vi "Configure Trigger (ZONE).vi"(4 "Enable Zone Qualified Trigger (F: Disable)":bool, 5 "Size and Location of Zone":T1={"Width of Zone (0 s)"=0.0, "Height of Zone (0 v)"=0.0, "X Center of Zone (0.0001 s)"=0.0001, "Y Center of Zone (0 v)"=5.0}, 6 "Zone State (F: Disable)":bool, 7 "Qualifying Condition (0: Must Intersect)":i32(ring) items=["Must Intersect", "Must Not Intersect"], 8 "error in (no error)":errorcluster, 9 "Zone Number (1: Zone 1)":i32(ring)=1 items=["Zone 1"=1, "Zone 2"=2], 10 "Analog Source Channel (0: Channel 1)":i32(ring) items=["Channel 1", "Channel 2", "Channel 3", "Channel 4"], 11 "VISA resource name":refnum<visa-resource-name>) -> (0 "error out":errorcluster, 3 "VISA resource name out":refnum<visa-resource-name>)   [LabVIEW 2015, in "Agilent 2000 3000 X-Series.lvlib"]
doc: "Configures the zone trigger mode. \n\nNote(s):\nThis VI is only applicable for Agilent InfiniiVision 4000 X-Series and 3000 T X-Series Oscilloscopes."
uses:
  <instrlib>/Agilent 2000 3000 X-Series/Agilent 2000 3000 X-Series.lvlib
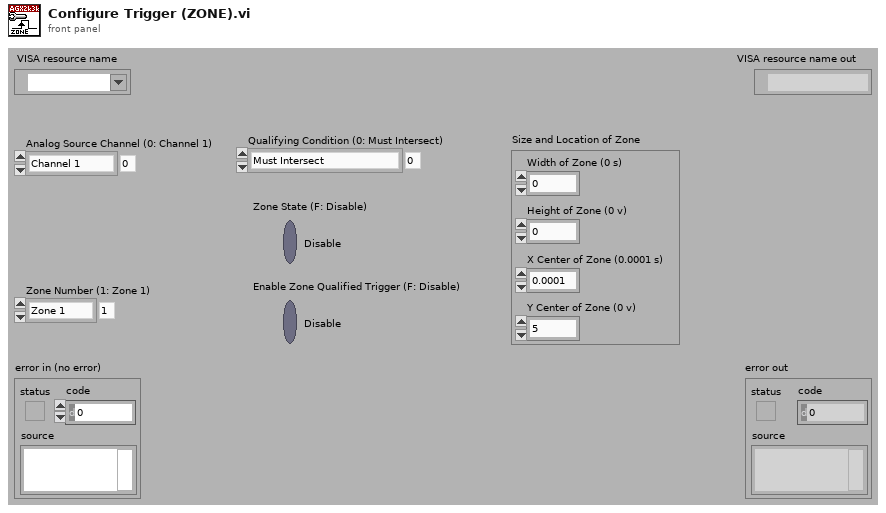
[diagram p1: front panel]
types:
  T1 = cluster{"Width of Zone (0 s)":dbl, "Height of Zone (0 v)":dbl, "X Center of Zone (0.0001 s)":dbl, "Y Center of Zone (0 v)":dbl}
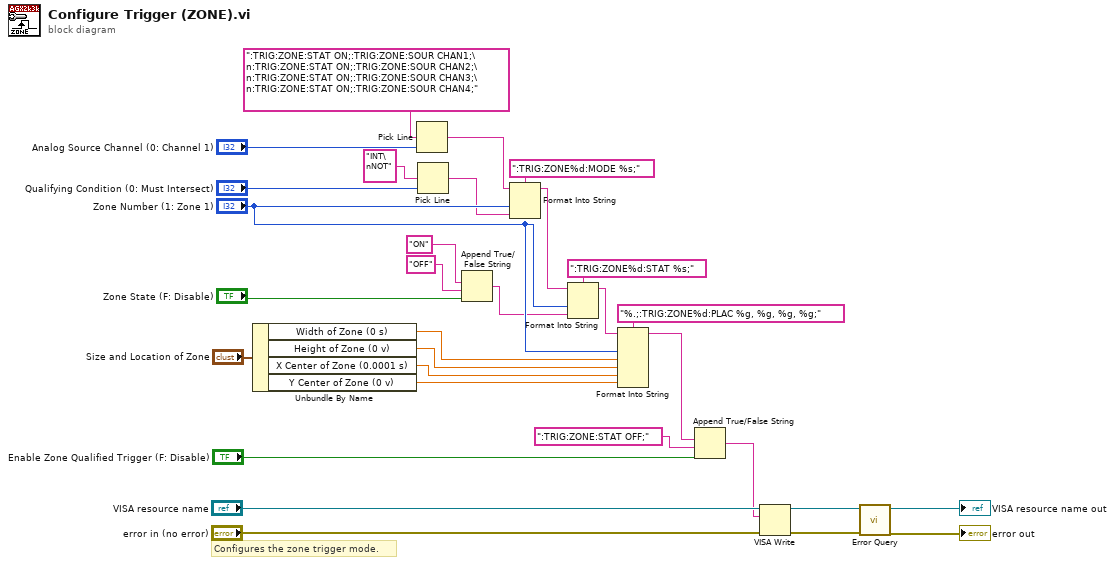
[diagram p0: block diagram]
diagram:
  # "Configures the zone trigger mode."
  n1 = Unbundle By Name("Size and Location of Zone") -> ("Width of Zone (0 s)"=w9:dbl, "Height of Zone (0 v)"=w8:dbl, "X Center of Zone (0.0001 s)"=w7:dbl, "Y Center of Zone (0 v)"=w6:dbl)
  n2 = Pick Line(multi-line string=":TRIG:ZONE:STAT ON;:TRIG:ZONE:SOUR CHAN1;\n:TRIG:ZONE:STAT ON;:TRIG:ZONE:SOUR CHAN2;\n:TRIG:ZONE:STAT ON;:TRIG:ZONE:SOUR CHAN3;\n:TRIG:ZONE:STAT ON;:TRIG:ZONE:SOUR CHAN4;", line index="Analog Source Channel (0: Channel 1)") -> (output string=w5:string)  [unwired: 1 out]
  n3 = Pick Line(multi-line string="INT\nNOT", line index="Qualifying Condition (0: Must Intersect)") -> (output string=w25:string)  [unwired: 1 out]
  n4 = Append True/False String(1:"Zone State (F: Disable)", 2:"OFF", 3:"ON") -> (0:w19:string)  [unwired: 1 out]
  n5 = Format Into String(format string=":TRIG:ZONE%d:MODE %s;", initial string=w5, "Zone Number (1: Zone 1)", w25) -> (resulting string=w21:string)  [unwired: 1 in, 1 out]
  n6 = Format Into String(format string=":TRIG:ZONE%d:STAT %s;", initial string=w21, "Zone Number (1: Zone 1)", w19) -> (resulting string=w18:string)  [unwired: 1 in, 1 out]
  n7 = Format Into String(format string="%.;:TRIG:ZONE%d:PLAC %g, %g, %g, %g;", initial string=w18, "Zone Number (1: Zone 1)", w9, w8, w7, w6) -> (resulting string=w2:string)  [unwired: 1 in, 1 out]
  n8 = Append True/False String(1:"Enable Zone Qualified Trigger (F: Disable)", 2:":TRIG:ZONE:STAT OFF;", 3:w2) -> (0:w1:string)  [unwired: 1 out]
  n9 = VISA Write(VISA resource name="VISA resource name", write buffer=w1, error in (no error)="error in (no error)") -> (VISA resource name out=w14:refnum<visa-resource-name>, error out=w13:errorcluster)  [unwired: 1 out]
  n10 = call <instrlib>:"Error Query.vi"("error in (no error)"=w13, "VISA resource name"=w14) -> ("error out"=→"error out":errorcluster, "VISA resource name out"=→"VISA resource name out":refnum<visa-resource-name>)  [unwired: 8 out]
